vi "MSScript_Format_FGen.vi"(9 "ValueArray":string[](array[string]), 10 "TagArray":string[](array[string]), 11 "MSScript in":refnum<class "MSScript.lvclass">) -> (0 "ValueErrorArray":bool[](array[boolean]), 1 "TagErrorArray":bool[](array[boolean]), 2 "ParamErrorArray":bool[](array[boolean]), 3 "Data":variant, 4 "#ofParamError":bool)   [LabVIEW 2018, in "MSScript.lvclass"]
uses:
  MSScript.lvclass
  Ctl/MSEditorParam FGen.ctl
  MSScript_Transform_Extended.vi
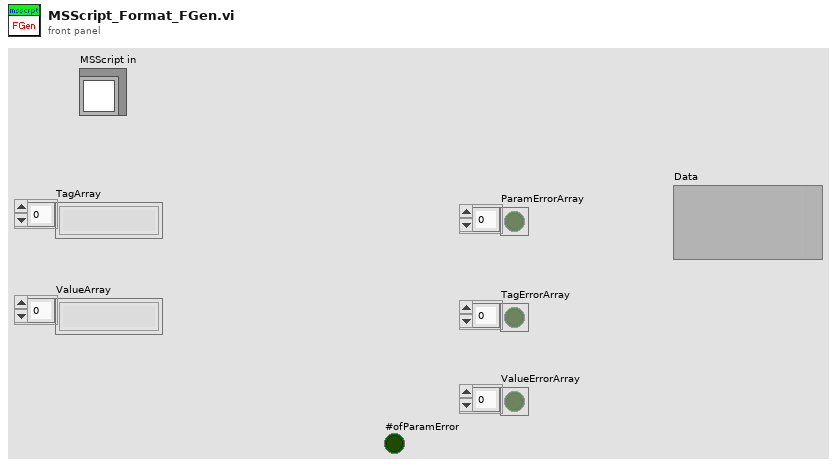
[diagram p1: front panel]
types:
  T1 = typedef "MSEditorParam FGen.ctl" = cluster{"amp":ext, "freq":ext}
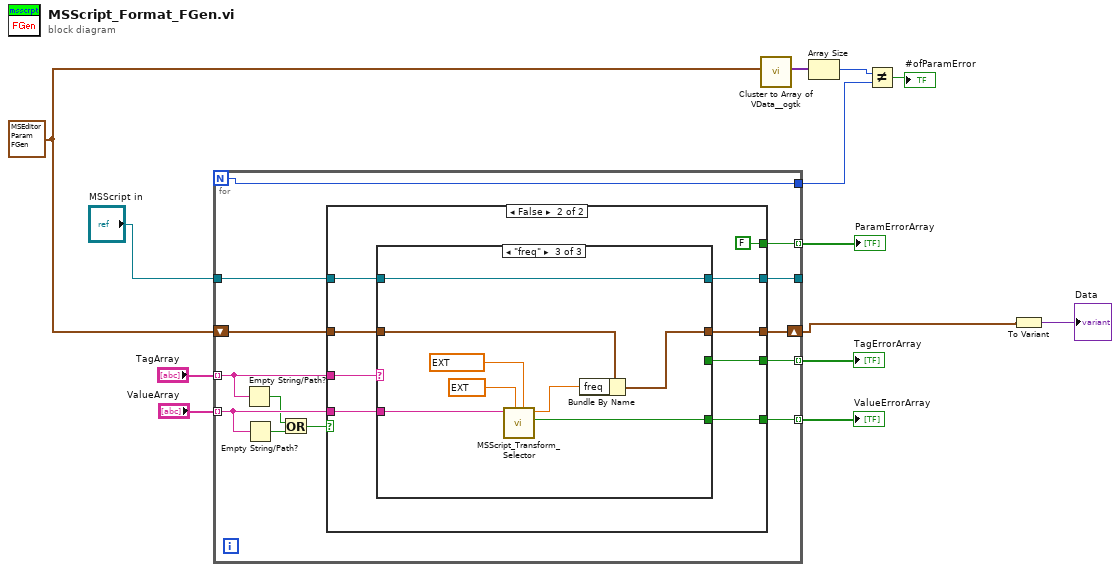
[diagram p0: block diagram]
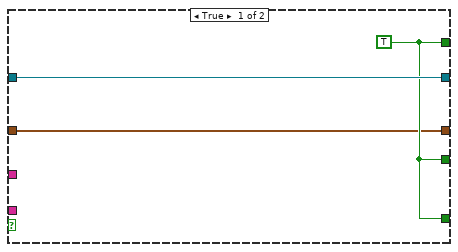
[diagram p2: hidden frame]
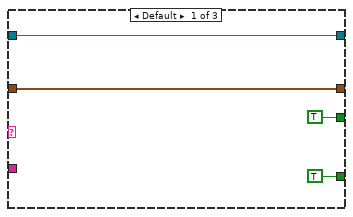
[diagram p3: hidden frame]
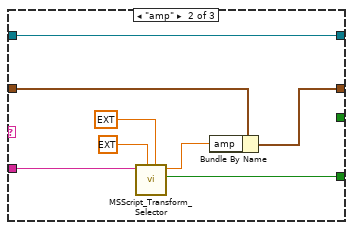
[diagram p4: hidden frame]
diagram:
  w4 = T1 {"amp"=0.001, "freq"=0.01} ("ParamValueType")
  n1 = for {
    N -> [w14]
    tunnel: "TagArray" -> [w22] mode=indexing
    tunnel: "ValueArray" -> [w21] mode=indexing
    tunnel: [w26] -> w11 mode=indexing
    tunnel: "MSScript in" -> [w25]
    tunnel: [w24] -> w10 mode=indexing
    tunnel: [w23] -> _
    tunnel: [w17] -> w9 mode=indexing
    shift-right: [w15] -> w2
    shift-left: w4 -> [w16]
    tunnel: [w14] -> w3
    n2 = Empty String/Path?(string/path=w22) -> (empty?=w19:bool)
    n3 = Empty String/Path?(string/path=w21) -> (empty?=w20:bool)
    n4 = Or(x=w19, y=w20) -> (x .or. y?=w18:bool)
    n5 = case shown="False" w18 {
      tunnel: [w28 w31] -> w26
      tunnel: w25 -> [w29 w37]
      tunnel: [w28 w30] -> w24
      tunnel: [w29 w33] -> w23
      tunnel: w22 -> [_ w35]
      tunnel: w21 -> [_ w34]
      tunnel: [w28 FALSE] -> w17
      tunnel: w16 -> [w27 w36]
      tunnel: [w27 w32] -> w15
      frame True {
        w28 = TRUE
      }
      frame False {
        n6 = case shown="\"freq\"" w35 {
          tunnel: [TRUE _ _] -> w31
          tunnel: w37 -> [w40 w47 w52]
          tunnel: w34 -> [_ w48 w56]
          tunnel: [TRUE ("Value Error?") w50 w58] -> w30
          tunnel: [w40 w47 w52] -> w33
          tunnel: w36 -> [w39 w45 w54]
          tunnel: [w39 w44 w53] -> w32
          frame Default {
          }
          frame "amp" {
            n7 = call-poly "MSScript_Transform_Selector.vi"("upper limit (Inf)"=ext 3.3 ("upper limit"), "lower limit (-Inf)"=ext 0.0 ("lower limit"), "Check_Str"=w48) -> ("Value Error?"=w50:bool, "Value Output"=w46:ext)  [unwired: 6 in, 1 out]
            n8 = Bundle By Name(cluster=w45, "amp"=w46) -> (w44:T1)
          }
          frame "freq" {
            n9 = call-poly "MSScript_Transform_Selector.vi"("upper limit (Inf)"=ext 2000000.0 ("upper limit"), "lower limit (-Inf)"=ext 0.00099999999999999999996 ("lower limit"), "Check_Str"=w56) -> ("Value Error?"=w58:bool, "Value Output"=w55:ext)  [unwired: 6 in, 1 out]
            n10 = Bundle By Name(cluster=w54, "freq"=w55) -> (w53:T1)
          }
        }
      }
    }
  }
  "TagErrorArray" <- w11
  "ValueErrorArray" <- w10
  "ParamErrorArray" <- w9
  n11 = call <userlib>:"Cluster to Array of VData__ogtk.vi"("Cluster"=w4) -> ("Array of VData"=w7:variant[])  [unwired: 9 in, 1 out]
  n12 = Array Size(array=w7) -> (size(s)=w6:i32)
  n13 = Not Equal?(x=w6, y=w3) -> (x != y?=→"#ofParamError":bool)
  n14 = To Variant(anything=w2) -> (Variant=→"Data":variant)
